vi "POST.vi"(8 "error in (no error)":errorcluster, 10 "SM_POST (Move to Diagnostics Tab)_UI":bool, 11 "ZenGage v3.0 UI in":refnum<class "ZenGage v3.0 UI.lvclass">) -> (0 "error out":errorcluster, 3 "ZenGage v3.0 UI out":refnum<class "ZenGage v3.0 UI.lvclass">)   [LabVIEW 2015, in "ZenGage v3.0 UI.lvclass"]
uses:
  ZenGage v3.0 UI.lvclass
  ZenGage v3.0 UI.lvclass/ZenGage v3.0 UI.ctl
  Type Definitions/General/UI States(UI button enable disable).ctl
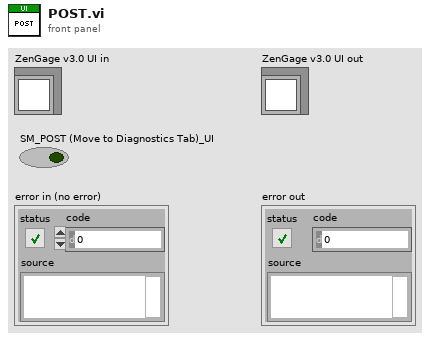
[diagram p1: front panel]
types:
  T1 = enum32{"Arduino Motor", "Sensor trigger", "Hardware Button", "Camera Optics"}
  T2 = typedef "ZenGage v3.0 UI.lvclass/UI States(UI button enable disable).ctl" = cluster{"Inspection":cluster{"Inspection States":enum16{"PreSelect", "Back _Inspection", "Analytics", "Ready To Run", "Ready To Insert", "Enable All buttons", "Disable All Buttons", "Settings", "Select", "Stop", "Pause", "Inspect"}}, "Diagnostics":cluster{"Diagnostics States":enum16{"Enable All", "Camera Optics Fail", "Loading Bar", "Camera Optics", "Motor", "Arduino", "POST Done", "POST"}}, "Edit Tolerance":cluster{"Edit Limits":enum16{"Update List"}, "Enable Disable Measurements":enum16{"Back to Edit Tolerance"}, "Page Select":enum16{"Edit Tolerance Limits", "Enable Disable Buttons"}}, "Page Select":enum16{"Edit Tolerance", "Diagnostics", "Inspection"}}
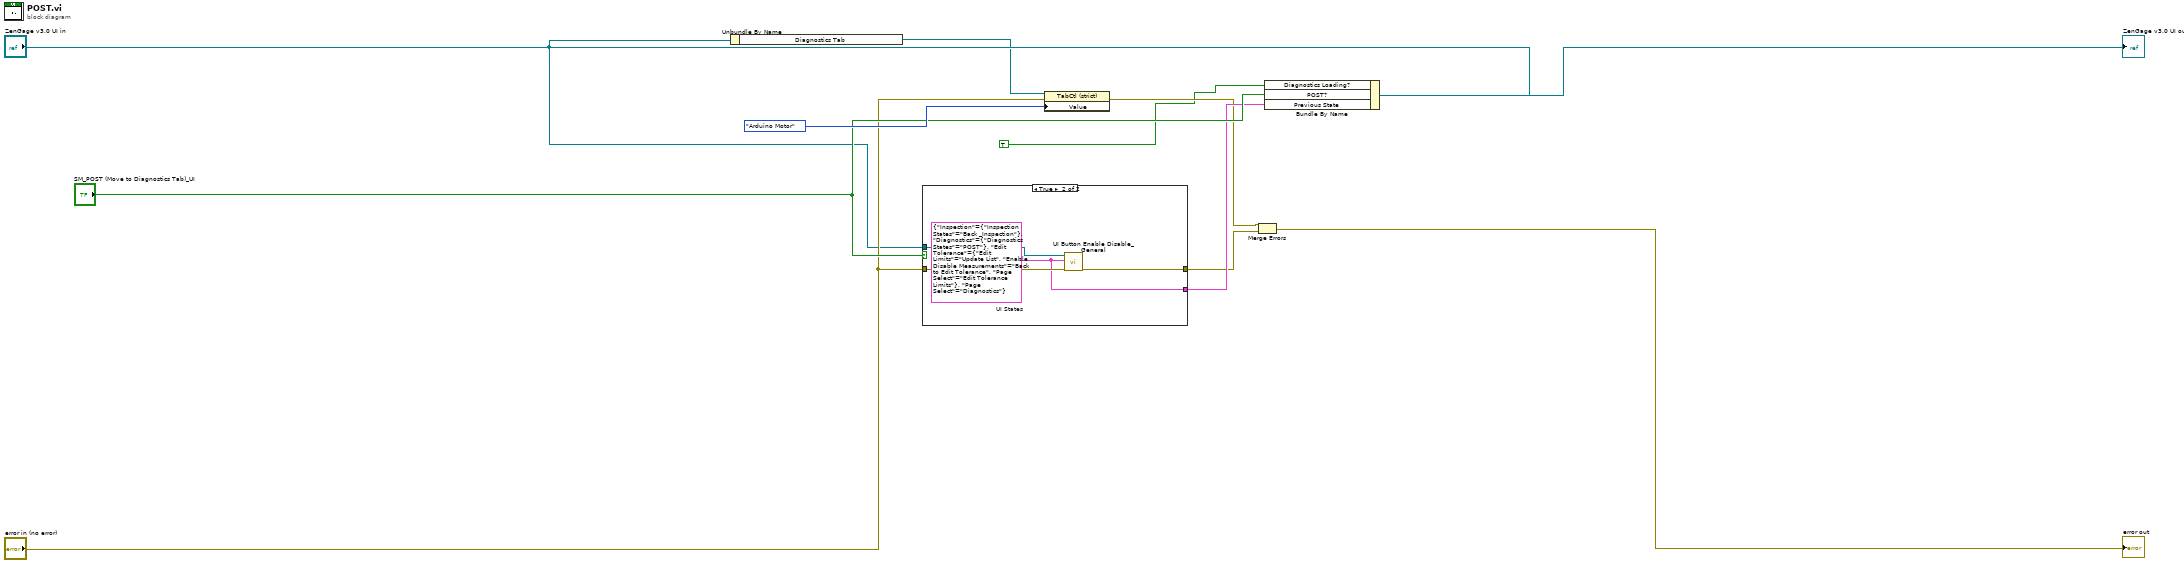
[diagram p0: block diagram]
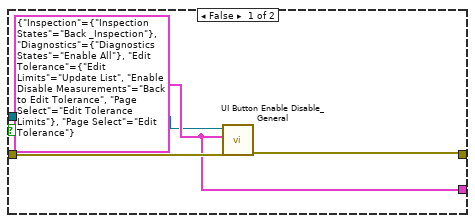
[diagram p2: hidden frame]
diagram:
  n1 = Unbundle By Name("ZenGage v3.0 UI in") -> ("Diagnostics Tab"=w1:refnum<vi>)
  n2 = case shown="True" "SM_POST (Move to Diagnostics Tab)_UI" {
    tunnel: "error in (no error)" -> [w15 w19]
    tunnel: [w14 w18] -> w5
    tunnel: [w13 w17] -> w8
    tunnel: "ZenGage v3.0 UI in" -> [w12 w16]
    frame False {
      w13 = T2 {"Inspection"={"Inspection States"=enum."Back _Inspection"}, "Diagnostics"={"Diagnostics States"=enum."Enable All"}, "Edit Tolerance"={"Edit Limits"=enum."Update List", "Enable Disable Measurements"=enum."Back to Edit Tolerance", "Page Select"=enum."Edit Tolerance Limits"}, "Page Select"=enum."Edit Tolerance"} ("UI States")
      n3 = call-dynamic "UI Button Enable Disable_General.vi"("error in (no error)"=w15, "UI States"=w13, "ZenGage v3.0 UI in"=w12) -> ("error out"=w14:errorcluster)  [unwired: 7 in, 1 out]
    }
    frame True {
      w17 = T2 {"Inspection"={"Inspection States"=enum."Back _Inspection"}, "Diagnostics"={"Diagnostics States"=enum."POST"}, "Edit Tolerance"={"Edit Limits"=enum."Update List", "Enable Disable Measurements"=enum."Back to Edit Tolerance", "Page Select"=enum."Edit Tolerance Limits"}, "Page Select"=enum."Diagnostics"}  # UI States
      n4 = call-dynamic "UI Button Enable Disable_General.vi"("error in (no error)"=w19, "UI States"=w17, "ZenGage v3.0 UI in"=w16) -> ("error out"=w18:errorcluster)  [unwired: 7 in, 1 out]
    }
  }
  n5 = property class="TabCtl (strict)"(reference=w1, error in="error in (no error)", "Value"=T1."Arduino Motor") -> (error out=w6:errorcluster)  [unwired: 1 out]
  n6 = Merge Errors(w6, w5) -> (→"error out":errorcluster)
  n7 = Bundle By Name(cluster="ZenGage v3.0 UI in", "Diagnostics Loading?"=TRUE ("Diagnostics.Diagnostics Loading?"), "POST?"="SM_POST (Move to Diagnostics Tab)_UI", "Previous State"=w8) -> (→"ZenGage v3.0 UI out":refnum<class "ZenGage v3.0 UI.lvclass">)
